vi "sound card.vi"(9 "f_c kHz":dbl=0.5, 10 "A_c V":dbl=1.0, 11 "k_f kHz/V":dbl=10.0) -> (5 "解调复原的基带信号":waveform(dbl)(graph))   [LabVIEW 2020]
uses:
  <vilib>/sound2/lvsound2.llb/Sampling Mode.ctl
  <vilib>/sound2/lvsound2.llb/Sound Data Format.ctl
  <vilib>/sound2/lvsound2.llb/Sound Output Write (DBL Single).vi
  <vilib>/sound2/lvsound2.llb/Sound Input Read (DBL).vi
  <vilib>/express/express shared/transition.llb/Dynamic To Waveform Array.vi
  <vilib>/express/express arith-compare/Formula/Block/exnFormulaBlock how many pts in the wave.vi
  <vilib>/express/express shared/ex_Modify Signal Name.vi
  <vilib>/express/express shared/transition.llb/Waveform Array To Dynamic.vi
  <vilib>/express/express analysis/Spectral/Block/exnSpectralBlock spectral measurements peak poly.vi
  <vilib>/express/express analysis/Spectral/Block/exnSpectralBlock spectral measurements peak DDT.vi
  <vilib>/express/express arith-compare/Formula/XNode/ExpressFormulaBlockNode.xnode
  <vilib>/express/express analysis/Spectral/XNode/ExpressSpectralMeasurementsBlockNode.xnode
  <vilib>/measure/NI_MABase.lvlib
  <vilib>/Analysis/NI_AALPro.lvlib
panel:
  in  "Input Device ID":u32
  in  "Output Device ID":u32
  in  "Stop":bool
  out "调制信号":waveform(dbl)[](graph)
  out "f_c Hz":dbl
  out "采样数":dbl
  out "采样率 Hz":dbl
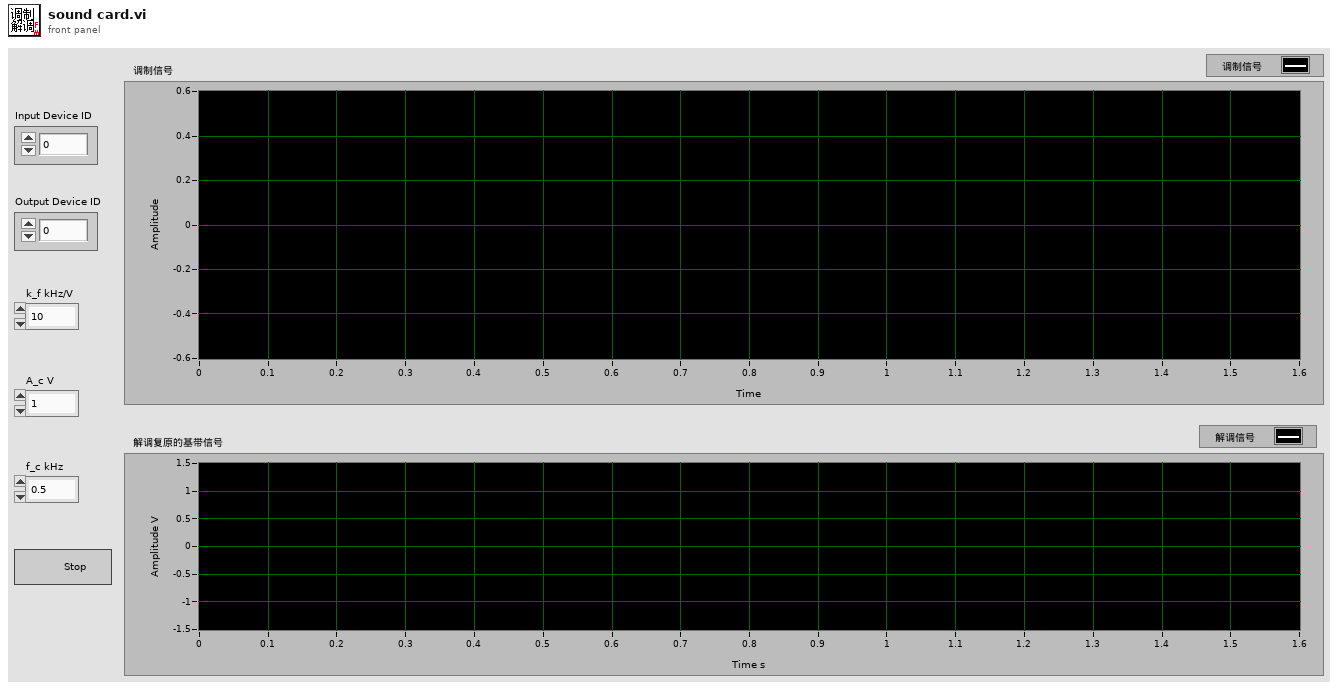
[diagram p1: front panel]
types:
  T1 = typedef "Sound Data Format.ctl" = cluster{"sample rate (S/s)":dbl, "number of channels":i32, "bits per sample":i32}
  T2 = typedef "Sampling Mode.ctl" = i32
  T3 = typedef "Sound Output Task ID.ctl" = u32
  T4 = typedef "Sound Input Task ID.ctl" = u32
  T5 = cluster{"averaging mode":u16, "weighting mode":u16, "number of averages":u32}
  T6 = cluster{"dB On (F)":bool, "unwrap phase (F)":bool, "convert to degree (F)":bool}
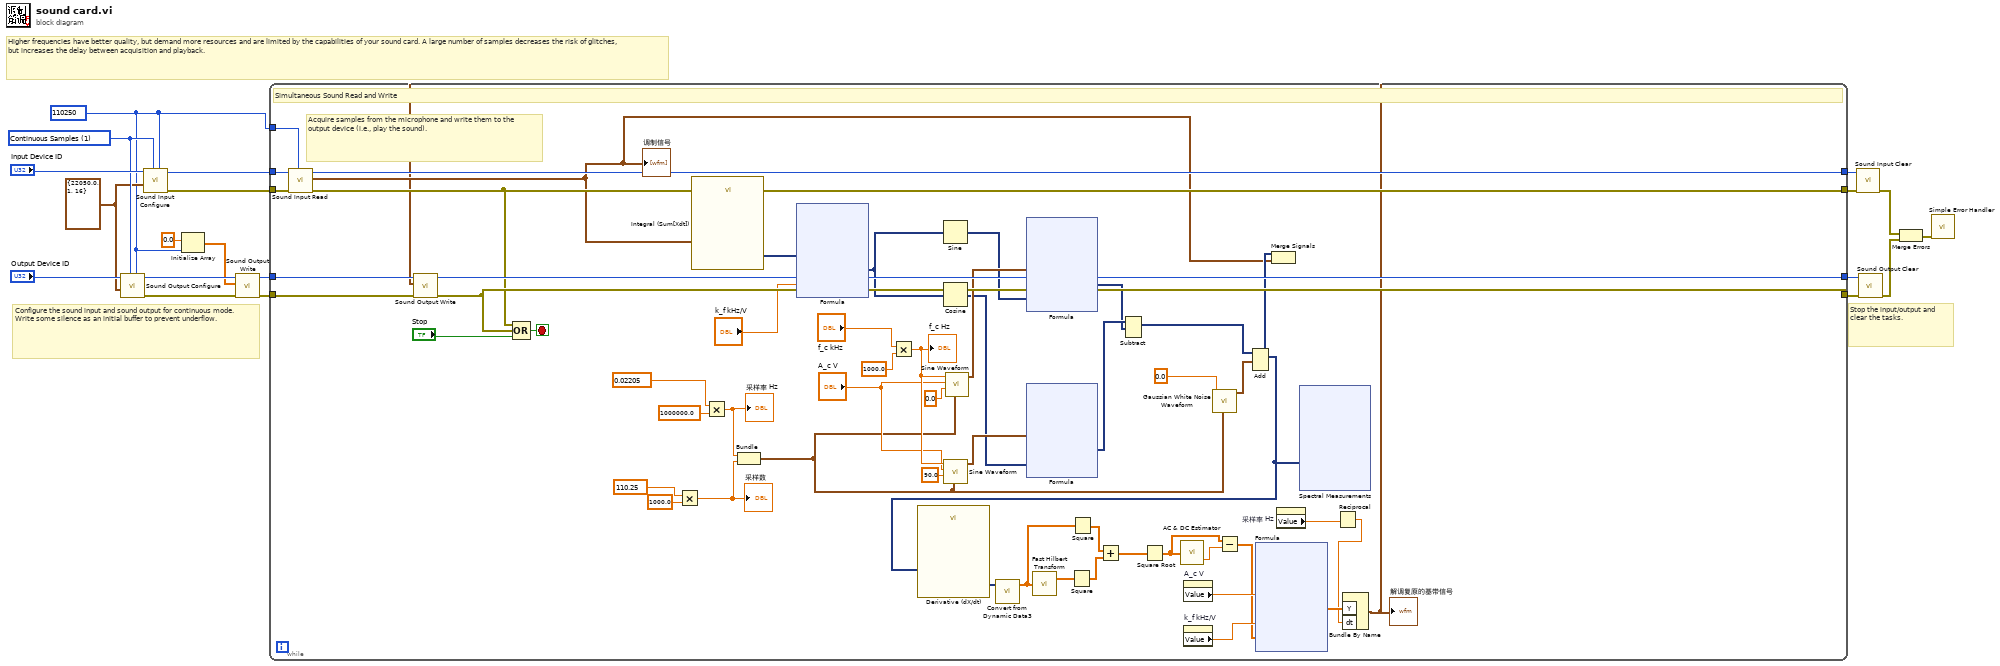
[diagram p0: block diagram]
diagram:
  w1 = 110250 ("Number of Samples/ch 2")
  w4 = T1 {"sample rate (S/s)"=22050.0, "number of channels"=1, "bits per sample"=16} ("Sound Format")
  w10 = T2 1 items=["Finite Samples", "Continuous Samples"] ("sample mode")
  # "Higher frequencies have better quality, but demand more resources and are limited by the capabilities of your sound card. A large number of samples decreases the risk of glitches, but increases the delay between acquisition and playback."
  # "Stop the input/output and clear the tasks."
  # "Configure the sound input and sound output for continuous mode. Write some silence as an initial buffer to prevent underflow."
  n1 = call <vilib>:"Sound Output Configure.vi"("number of samples/ch"=w1, "sample mode"=w10, "sound format"=w4, "device ID"="Output Device ID") -> ("error out"=w8:errorcluster, "task ID"=w9:T3)  [unwired: 6 in]
  n2 = call <vilib>:"Sound Input Configure.vi"("number of samples/ch"=w1, "sample mode"=w10, "sound format"=w4, "device ID"="Input Device ID") -> ("error out"=w12:errorcluster, "task ID"=w11:T4)  [unwired: 6 in]
  n3 = Initialize Array(0.0 ("element"), w1) -> (w2:dbl[])
  n4 = call-poly <vilib>:"Sound Output Write.vi"("error in (no error)"=w8, "data"=w2, "task ID"=w9) -> ("error out"=w7:errorcluster, "task ID out"=w6:T3)  [unwired: 7 in]
  n5 = while {
    tunnel: w1 -> [w69]
    tunnel: w11 -> [w71]
    tunnel: [w68] -> w15
    tunnel: w6 -> [w72]
    tunnel: [w70] -> w18
    tunnel: w7 -> [w67]
    tunnel: [w64] -> w19
    tunnel: w12 -> [w73]
    tunnel: [w63] -> w20
    stop <- w65 stop-if-true
    # "Acquire samples from the microphone and write them to the output device (i.e., play the sound)."
    # "Simultaneous Sound Read and Write"
    n6 = call-poly <vilib>:"Sound Input Read.vi"("number of samples/ch"=w69, "error in (no error)"=w73, "task ID"=w71) -> ("error out"=w63:errorcluster, "data"=w24:waveform(dbl)[], "task ID out"=w68:T4)  [unwired: 6 in]
    "调制信号" <- w24
    n7 = Multiply(x=110.25 ("采样数 k"), y=1000.0) -> (x*y=w37:dbl)
    "采样数" <- w37
    n8 = call "Integral (Sum[Xdt])"("Signals"=w24) -> ("Result"=w46:dynamicdata)  [unwired: 5 in, 1 out]
    n9 = Multiply(x=0.02205 ("采样率 MHz"), y=1000000.0) -> (x*y=w35:dbl)
    "采样率 Hz" <- w35
    n10 = Bundle(w35, w37) -> (w22:cluster{dbl, dbl})  [unwired: 1 in]
    n11 = xnode "Formula"("积分后的信号"=w46, "k_f"="k_f kHz/V") -> ("Result"=w61:dynamicdata)  [unwired: 1 in, 1 out]
    n12 = Multiply(x="f_c kHz", y=1000.0) -> (x*y=w33:dbl)
    "f_c Hz" <- w33
    n13 = Sine(x=w61) -> (sin(x)=w39:dynamicdata)
    n14 = Cosine(x=w61) -> (cos(x)=w38:dynamicdata)
    n15 = call <vilib>:"Sine Waveform.vi"("sampling info"=w22, "phase"=90.0, "amplitude"="A_c V", "frequency"=w33) -> ("signal out"=w41:waveform(dbl))  [unwired: 6 in, 1 out]
    n16 = call <vilib>:"Sine Waveform.vi"("sampling info"=w22, "phase"=0.0, "amplitude"="A_c V", "frequency"=w33) -> ("signal out"=w40:waveform(dbl))  [unwired: 6 in, 1 out]
    n17 = xnode "Formula"("sin载波"=w40, "sin相偏"=w39) -> ("Result"=w42:dynamicdata)  [unwired: 1 in, 1 out]
    n18 = xnode "Formula"("cos载波"=w41, "cos相偏"=w38) -> ("Result"=w62:dynamicdata)  [unwired: 1 in, 1 out]
    n19 = Subtract(1:w42, 2:w62) -> (0:w44:dynamicdata)  [unwired: 1 in, 1 out]
    n20 = property on="A_c V" class="DigNum (strict)"() -> ("Value"=w57:dbl)  [unwired: 2 in, 2 out]
    n21 = property on="k_f kHz/V" class="DigNum (strict)"() -> ("Value"=w58:dbl)  [unwired: 2 in, 2 out]
    n22 = call <vilib>:"Gaussian White Noise Waveform.vi"("sampling info"=w22, "standard deviation"=0.0 ("标准差 V")) -> ("signal out"=w45:waveform(dbl))  [unwired: 8 in, 1 out]
    n23 = Add(1:w45, 2:w44) -> (0:w60:dynamicdata)  [unwired: 1 in, 1 out]
    n24 = call "Derivative (dX/dt)"("Signals"=w60) -> ("Result"=w52:dynamicdata)  [unwired: 5 in, 1 out]
    n25 = call "Convert from Dynamic Data3"("Dynamic Data Type"=w52) -> ("Array"=w47:dbl[])  [unwired: 3 in]
    n26 = call <vilib>:"Fast Hilbert Transform.vi"("X"=w47) -> ("Hilbert{X}"=w48:dbl[])  [unwired: 1 out]
    n27 = Square(x=w48) -> (x^2=w50:dbl[])
    n28 = Square(x=w47) -> (x^2=w49:dbl[])
    n29 = Add(x=w49, y=w50) -> (x+y=w51:dbl[])
    n30 = Square Root(x=w51) -> (sqrt(x)=w53:dbl[])
    n31 = call <vilib>:"AC & DC Estimator.vi"("Signal (V)"=w53) -> ("DC estimate (V)"=w55:dbl)  [unwired: 1 out]
    n32 = Subtract(x=w53, y=w55) -> (x-y=w56:dbl[])
    n33 = xnode "Formula"("A_c"=w57, "k_f"=w58, "Signals"=w56) -> ("Result"=w59:dbl[])  [unwired: 1 in, 1 out]
    n34 = Merge Signals(w60, w24) -> ()  [unwired: 1 out]
    n35 = property on="采样率 Hz" class="DigNum (strict)"() -> ("Value"=w54:dbl)  [unwired: 2 in, 2 out]
    n36 = xnode "Spectral Measurements"("Signals"=w60) -> ()  [unwired: 1 in, 3 out]
    n37 = Reciprocal(x=w54) -> (1/x=w21:dbl)
    n38 = Bundle By Name("Y"=w59, "dt"=w21) -> (w23:waveform(dbl))  [unwired: 1 in]
    "解调复原的基带信号" <- w23
    n39 = call-poly <vilib>:"Sound Output Write.vi"("error in (no error)"=w67, "data"=w23, "task ID"=w72) -> ("error out"=w64:errorcluster, "task ID out"=w70:T3)  [unwired: 7 in]
    n40 = Compound Arithmetic op=OR(w63, w64, "Stop") -> (w65:bool)
  }
  n41 = call <vilib>:"Sound Input Clear.vi"("error in (no error)"=w20, "task ID"=w15) -> ("error out"=w13:errorcluster)  [unwired: 9 in]
  n42 = call <vilib>:"Sound Output Clear.vi"("error in (no error)"=w19, "task ID"=w18) -> ("error out"=w14:errorcluster)  [unwired: 9 in]
  n43 = Merge Errors(w13, w14) -> (w5:errorcluster)
  n44 = call <vilib>:"Simple Error Handler.vi"("error in (no error)"=w5) -> ()  [unwired: 4 in, 5 out]
